vi "CANSAT.vi"() -> ()   [LabVIEW 2017]
panel:
  out "?":dbl
  out "?":dbl
  out "?":dbl
  out "?":dbl
  out "?":dbl
  out "?":dbl
  out "?":dbl
  out "?":dbl
  out "?":dbl[](graph)
  out "?":dbl[](graph)
  out "?":dbl[](graph)
  out "?":dbl[](graph)
  out "?":dbl[](graph)
  out "PRESSURE":dbl(knob) scale=0.0..10.0
  out "?":dbl[](graph)
  out "?":dbl
  out "?":dbl
  in  "?":bool
  in  "?":bool
  out "SHOTS":dbl
  in  "?":bool
  out "?":dbl
  out "?":dbl
  out "?":dbl
  out "?":dbl[](graph)
  in  "VOLTAGE":dbl(slide) scale=0.0..10.0
  in  "TEMPERATURE":dbl(slide) scale=0.0..100.0
  out "?":bool
  out "?":bool
  out "?":bool
  out "?":bool
  out "?":bool
  out "?":bool
  out "?":bool
  out "?":dbl
  out "?":dbl format="%<%H:%M>t"
  out "?":dbl
  out "?":string(combo)
  out "?":dbl
  # "TEAM ID"
  # "SOFTWARE STATE"
  # "LAUNCH WAIT"
  # "MISSION \nTIME"
  # "ASCENT"
  # "PACKET\nCOUNT"
  # "ROCKET\nDEPLOYMENT"
  # "TEMPERATURE"
  # "SOFTWARE STATE"
  # "PRESSURE"
  # "STABILIZATION"
  # "CONNECTION DETAILS"
  # "VOLTAGE"
  # "SEPARATION"
  # "ALTITUDE"
  # "COM PORT"
  # "DESCENT"
  # "GPS TIME"
  # "PITCH"
  # "BAUD RATE"
  # "LANDED"
  # "GPS LATITUDE"
  # "ROLL"
  # "CAMERA"
  # "BUTTONS"
  # "GPS LONGITUDE"
  # "BLADE RPM"
  # "GPS ALTITUDE"
  # "GPS SATS"
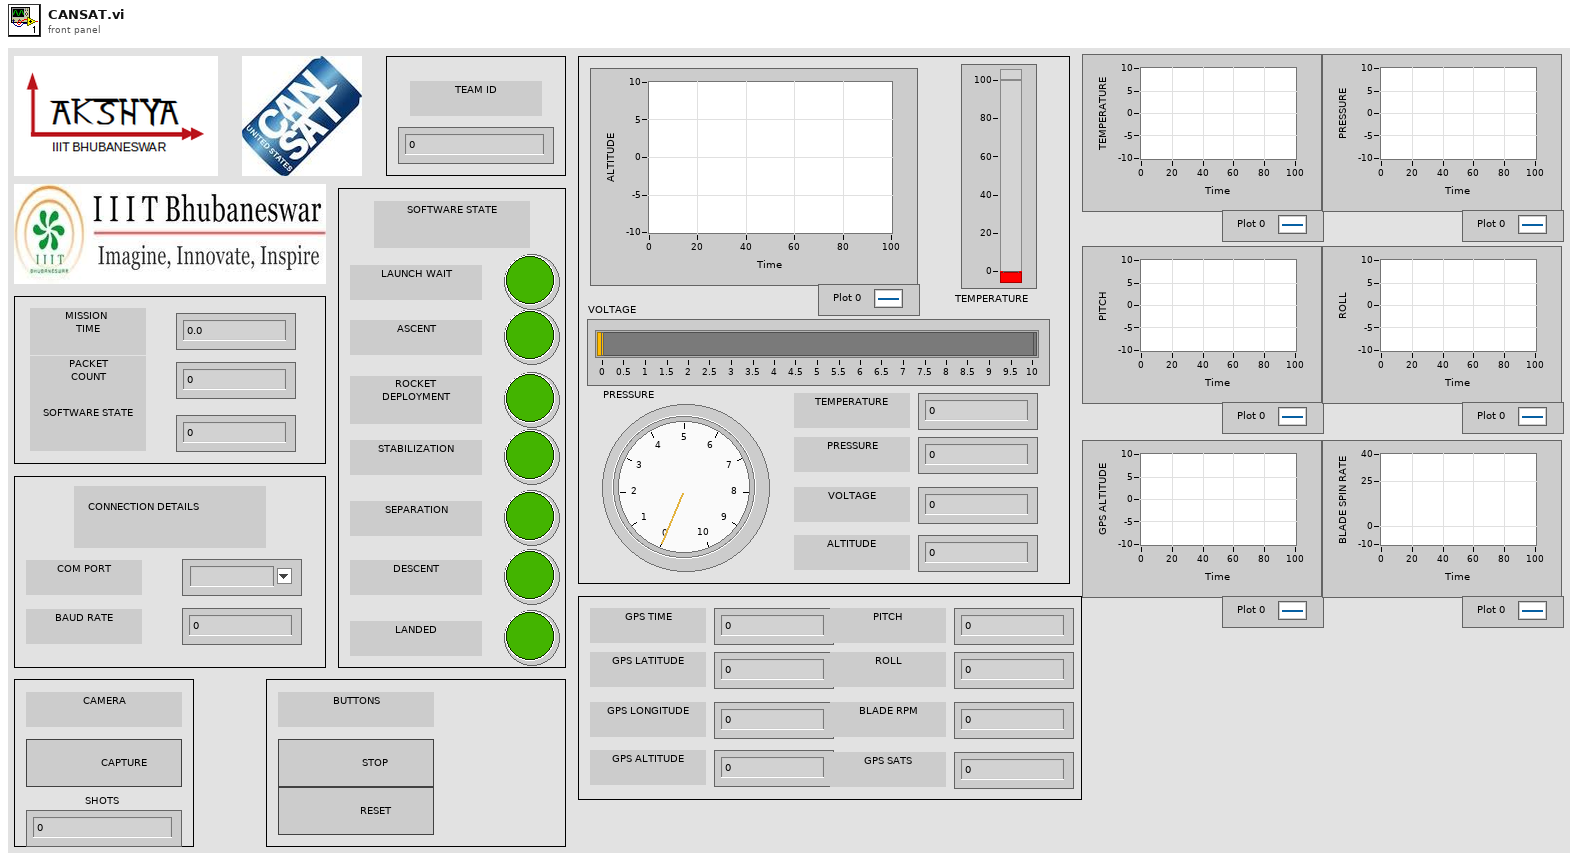
[diagram p1: front panel]
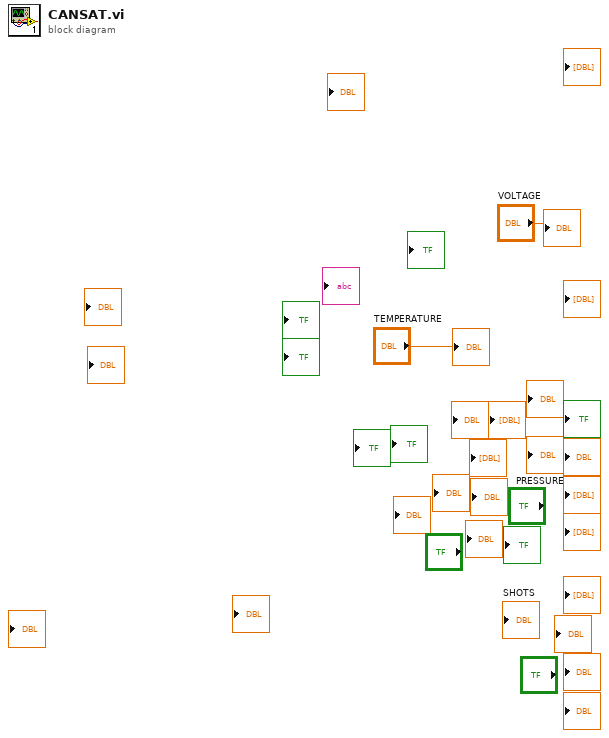
[diagram p0: block diagram]
diagram:
  "?" <- "VOLTAGE"
  "?" <- "TEMPERATURE"
